vi "PulseCal.vi"() -> ()   [LabVIEW 2022 SP3]
uses:
  <vilib>/Utility/file.llb/Write To Spreadsheet File (DBL).vi
  -CalTransducer/Hydros.ctl
panel:
  in  "scope scale peak (V)":dbl=0.2 format="%.2f"
  in  "Hydrophone":T1
  out "Pulse Parameters":T2 {"focal length (cm)" format="%.2f"; "MI" format="%.2f"; "Ita.3" format="%.2f"; "Temporal Av Intensity \n(Ita mW/cm^2)" format="%.2f"; "Ipa.3" format="%.2f"; "Pulse Av Intensity\n (Ipa W/cm^2)" format="%.2f"; "Pulse Int \nIntegral (PII J/cm^2)" format="%.4e"; "pulse dur (Pd s)" format="%.2e"; "p.3" format="%.3f"; "neg peak pressure (MPa)" format="%.2f"; "derating (.3) factor" format="%.3f"; "prf" format="%.2f"; "Frequency (MHz)" format="%.2f"}
  in  "dig delay (micros)":dbl format="%.2f"
  in  "prf":dbl=1000.0 format="%.2f"
  out "window duration (s)":dbl format="%.2e"
  out "Line":dbl[](graph)
  in  "Line #":i32
  in  "Header format":u16(ring) items=["Riverside Format", "Ron Linear"]
  in  "new file path":path=path "C:/WINDOWS/DESKTOP/rri.eye"
  in  "Frequency (MHz)":dbl format="%.2f"
  # "This program is now obsolete. Nearly duplicated by BeamCal"
  # "Data is normalized to value of negative peak pressure"
  # "© 2000,2001 Riverside Research Institute"
  # "Highlight area to integrate. Left Yellow, Right Red."
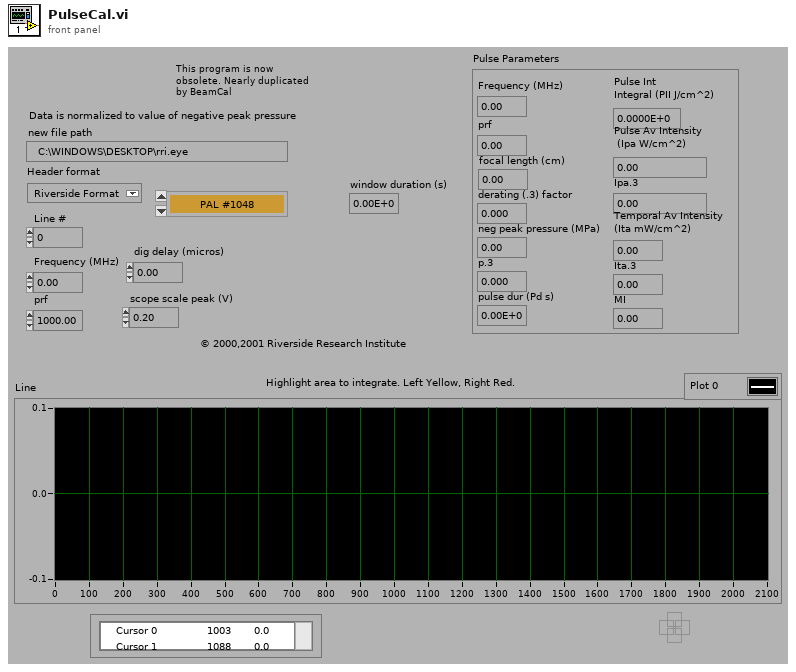
[diagram p1: front panel]
types:
  T1 = typedef "Hydros.ctl" = enum16{"PAL #1048", "PAL #525", "PAL #430a", "PAL #192", "DEAD PAL # 1403", "LOST UHI Onda", "DEAD PAL #1818", "PAL #1974", "DEAD #2266 w/booster", "PAL #2524 w/booster", "PAL FP21-20T", "PAL FP160-13  ", "PAL FP141-20", "PAL FP158-08T"}
  T2 = cluster{"Frequency (MHz)":dbl, "prf":dbl, "focal length (cm)":dbl, "derating (.3) factor":dbl, "neg peak pressure (MPa)":dbl, "p.3":dbl, "pulse dur (Pd s)":dbl, "Pulse Int \nIntegral (PII J/cm^2)":dbl, "Pulse Av Intensity\n (Ipa W/cm^2)":dbl, "Ipa.3":dbl, "Temporal Av Intensity \n(Ita mW/cm^2)":dbl, "Ita.3":dbl, "MI":dbl}
  T3 = cluster{"Name":string, "Color":u32, "Style":u8, "Point Style":u8, "Name Visible":bool, "Allow Drag":bool, "Lock Style":u32, "Plot":u32, "Index":i32, "Position":cluster{"X":dbl, "Y":dbl}}[]
  T4 = cluster{"Name":string, "Color":u32, "Style":u8, "Point Style":u8, "Name Visible":bool, "Allow Drag":bool, "Lock Style":u32, "Plot":u32, "Index":i32, "Position":cluster{"X":dbl, "Y":dbl}}
  T5 = cluster{"pulse dur (Pd s)":dbl, "Temporal Av Intensity \n(Ita mW/cm^2)":dbl, "Pulse Av Intensity\n (Ipa W/cm^2)":dbl, "Pulse Int \nIntegral (PII J/cm^2)":dbl}
  T6 = cluster{"Frequency (MHz)":dbl, "prf":dbl, "focal length (cm)":dbl, "derating (.3) factor":dbl, "neg peak pressure (MPa)":dbl, "pos peak pressure (MPa)":dbl, "p.3":dbl, "pulse dur (Pd s)":dbl, "Pulse Int \nIntegral (PII J/cm^2)":dbl, "Pulse Av Intensity\n (Ipa W/cm^2)":dbl, "Ipa.3":dbl, "Temporal Av Intensity \n(Ita mW/cm^2)":dbl, "Ita.3":dbl, "MI":dbl}
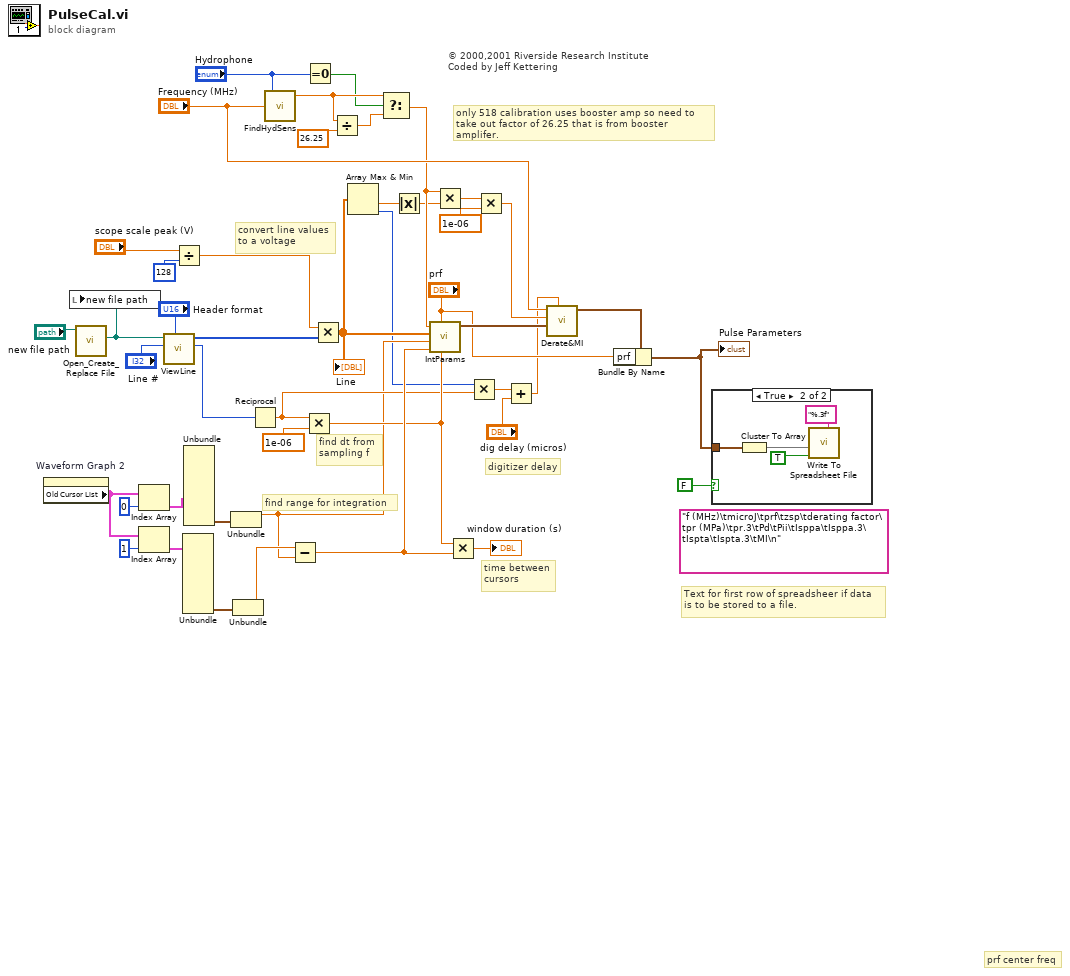
[diagram p0: block diagram]
diagram:
  (unwired) "f (MHz)\tmicroJ\tprf\tzsp\tderating factor\tpr (MPa)\tpr.3\tPd\tPii\tIsppa\tIsppa.3\tIspta\tIspta.3\tMI\n"
  # "digitizer delay"
  # "only 518 calibration uses booster amp so need to take out factor of 26.25 that is from booster amplifer."
  # "© 2000,2001 Riverside Research Institute\nCoded by Jeff Kettering"
  # "Text for first row of spreadsheer if data\nis to be stored to a file."
  # "prf center freq"
  # "convert line values\nto a voltage"
  # "time between\ncursors"
  # "find range for integration"
  # "find dt from\nsampling f"
  n1 = property on="Waveform Graph 2" class="WFGraph (strict)"() -> ("Old Cursor List"=w32:T3)  [unwired: 2 in, 2 out]
  n2 = call <vilib>:"Open_Create_Replace File.vi"("file path"="new file path") -> ("new file path"=w23:path)  [unwired: 5 in, 5 out]
  n3 = local write "new file path"(w23) -> ()
  n4 = Index Array(array=w32, index=0 ("Index")) -> (element=w42:T4)
  n5 = Index Array(array=w32, index=1 ("Index")) -> (element=w41:T4)
  n6 = call "ViewLine.vi"("Header format"="Header format", "Line #"="Line #", "new file path"=w23) -> ("sample rate MHz"=w37:u16, "Waveform Graph"=w3:i16[])  [unwired: 7 out]
  n7 = Divide(x="scope scale peak (V)", y=128) -> (x/y=w4:dbl)
  n8 = Unbundle(w41) -> ("Position"=w39:cluster{"X":dbl, "Y":dbl})  [unwired: 9 out]
  n9 = Unbundle(w42) -> ("Position"=w40:cluster{"X":dbl, "Y":dbl})  [unwired: 9 out]
  n10 = Unbundle(w40) -> ("X"=w6:dbl)  [unwired: 1 out]
  n11 = Unbundle(w39) -> ("X"=w38:dbl)  [unwired: 1 out]
  n12 = Reciprocal(x=w37) -> (1/x=w7:dbl)
  n13 = call "FindHydSens.vi"("Frequency (MHz)"="Frequency (MHz)", "Hydrophone"="Hydrophone") -> ("Sensitivity in Pa/V"=w17:dbl)  [unwired: 1 in, 2 out]
  n14 = Subtract(x=w38, y=w6) -> (x-y=w31:dbl)
  n15 = Multiply(x=w7, y=1e-06 ("x")) -> (x*y=w8:dbl)
  n16 = Equal To 0?(x="Hydrophone") -> (x = 0?=w16:bool)
  n17 = Multiply(x=w4, y=w3) -> (x*y=w13:dbl[])
  "Line" <- w13
  n18 = Divide(x=w17, y=26.25) -> (x/y=w20:dbl)
  n19 = Array Max & Min(array=w13) -> (min value=w12:dbl, min index (indices)=w5:i32)  [unwired: 2 out]
  n20 = Select(t=w17, s=w16, f=w20) -> (s? t:f=w15:dbl)
  n21 = Absolute Value(x=w12) -> (abs(x)=w2:dbl)
  n22 = call "IntParams.vi"("sample interval (s/Pt)"=w8, "prf"="prf", "Length of Subset"=w31, "Index of subset"=w6, "Data"=w13, "Sens"=w15) -> ("Intensity Variables"=w28:T5)  [unwired: 5 out]
  n23 = Multiply(x=w15, y=w2) -> (x*y=w34:dbl)
  n24 = Multiply(x=w8, y=w31) -> (x*y=→"window duration (s)":dbl)
  n25 = Multiply(x=w5, y=w7) -> (x*y=w11:dbl)
  n26 = Multiply(x=w34, y=1e-06 ("x")) -> (x*y=w30:dbl)
  n27 = Add(x=w11, y="dig delay (micros)") -> (x+y=w9:dbl)
  n28 = call "Derate&MI.vi"("Frequency (MHz)"="Frequency (MHz)", "neg peak pressure (MPa)"=w30, "Intensity Variables"=w28, "delay (ms)"=w9) -> ("Pulse Parameters"=w27:T6)  [unwired: 2 in, 4 out]
  n29 = Bundle By Name(cluster=w27, "prf"="prf") -> (w22:T6)
  "Pulse Parameters" <- w22
  n30 = case shown="True" FALSE ("Case Constant\n(See Context Help)") {
    tunnel: w22 -> [_ w49]
    frame False {
    }
    frame True {
      n31 = Cluster To Array(cluster=w49) -> (array=w47:dbl[])
      n32 = call-poly <vilib>:"Write To Spreadsheet File.vi"("format (%.3f)"="%.3f" ("format string"), "append to file? (new file:F)"=TRUE, "1D data"=w47) -> ()  [unwired: 3 in, 3 out]
    }
  }
